vi "LaunchEquations.vi"(7 "Finding V?":bool, 8 "Y (feet)":dbl=8.0, 9 "X (feet)":dbl, 10 "V (m/s)":dbl=14.5, 11 "Angle (degrees)":dbl) -> (2 "V (m/s)":dbl, 3 "Angle (degrees)":dbl)   [LabVIEW 2015]
panel:
  out "Drag (m/s^2)":dbl
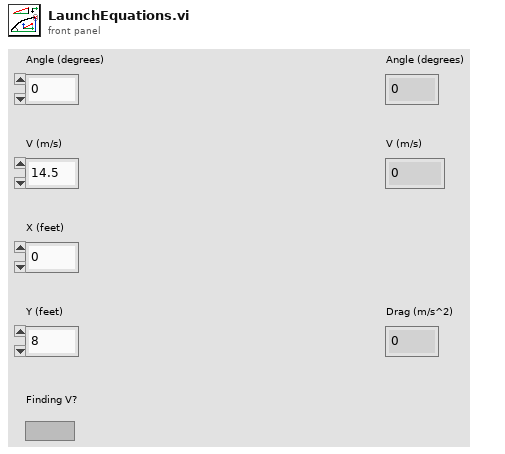
[diagram p1: front panel]
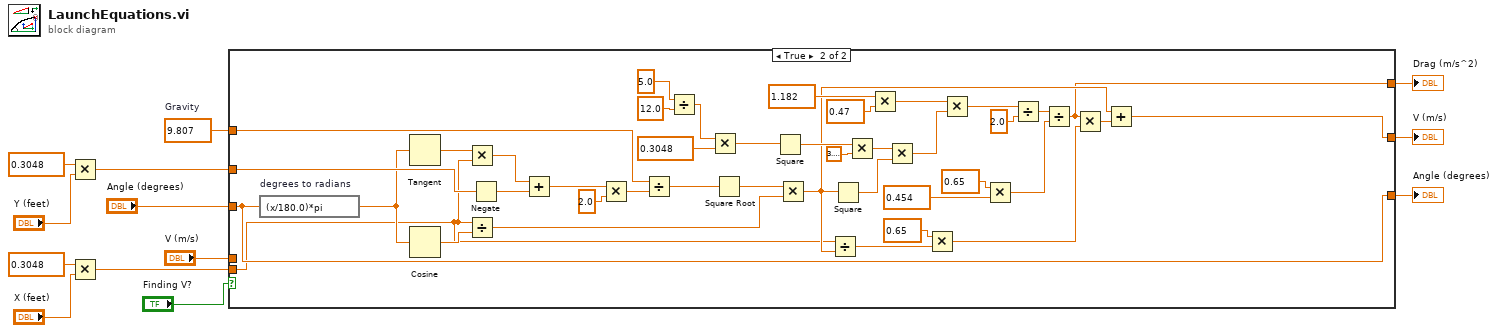
[diagram p0: block diagram]
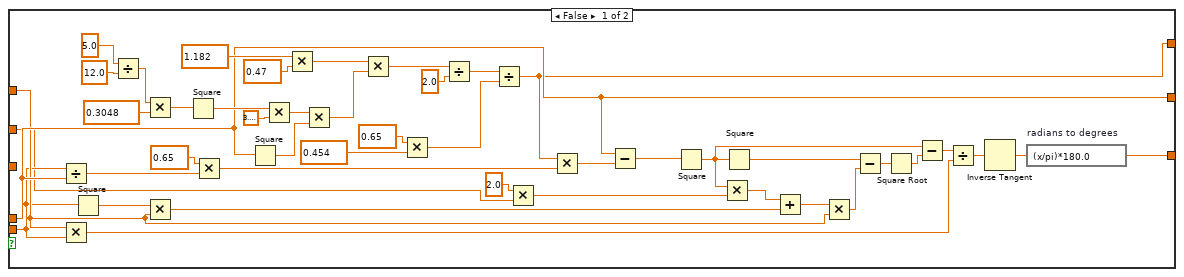
[diagram p2: hidden frame]
diagram:
  w7 = 9.807  # Gravity
  n1 = Multiply(x=0.3048, y="Y (feet)") -> (x*y=w1:dbl)
  n2 = Multiply(x=0.3048, y="X (feet)") -> (x*y=w4:dbl)
  n3 = case shown="True" "Finding V?" {
    tunnel: w4 -> [w16 w60]
    tunnel: "V (m/s)" -> [w18 _]
    tunnel: "Angle (degrees)" -> [_ w89]
    tunnel: [w19 w89] -> w10
    tunnel: [w18 w65] -> w9
    tunnel: [w14 w59] -> w8
    tunnel: w7 -> [w17 w94]
    tunnel: w1 -> [w15 w99]
    frame False {
      n4 = Divide(x=w16, y=w18) -> (x/y=w22:dbl)
      n5 = Multiply(x=w17, y=w16) -> (x*y=w47:dbl)
      n6 = Square(x=w16) -> (x^2=w58:dbl)
      n7 = Divide(x=5.0 ("Radius (in)"), y=12.0 ("Inches-feet")) -> (x/y=w31:dbl)
      n8 = Multiply(x=w31, y=0.3048 ("Feet-meters")) -> (x*y=w30:dbl)
      n9 = Multiply(x=w58, y=w17) -> (x*y=w55:dbl)
      n10 = Square(x=w30) -> (x^2=w42:dbl)
      n11 = Multiply(x=0.65 ("Drag approximation"), y=w22) -> (x*y=w21:dbl)
      n12 = Square(x=w18) -> (x^2=w40:dbl)
      n13 = Multiply(x=w42, y=3.141592653589793) -> (x*y=w41:dbl)
      n14 = Multiply(x=1.182 ("Air density"), y=0.47 ("Drag coefficient")) -> (x*y=w38:dbl)
      n15 = Multiply(x=w41, y=w40) -> (x*y=w39:dbl)
      n16 = Multiply(x=w38, y=w39) -> (x*y=w37:dbl)
      n17 = Multiply(x=0.65 ("Mass (lbs)"), y=0.454 ("Lbs-kgs")) -> (x*y=w26:dbl)
      n18 = Divide(x=w37, y=2.0) -> (x/y=w28:dbl)
      n19 = Divide(x=w28, y=w26) -> (x/y=w14:dbl)
      n20 = Multiply(x=2.0, y=w15) -> (x*y=w56:dbl)
      n21 = Multiply(x=w14, y=w21) -> (x*y=w24:dbl)
      n22 = Subtract(x=w18, y=w24) -> (x-y=w23:dbl)
      n23 = Square(x=w23) -> (x^2=w44:dbl)
      n24 = Multiply(x=w44, y=w56) -> (x*y=w54:dbl)
      n25 = Square(x=w44) -> (x^2=w52:dbl)
      n26 = Add(x=w54, y=w55) -> (x+y=w53:dbl)
      n27 = Multiply(x=w53, y=w17) -> (x*y=w51:dbl)
      n28 = Subtract(x=w52, y=w51) -> (x-y=w50:dbl)
      n29 = Square Root(x=w50) -> (sqrt(x)=w49:dbl)
      n30 = Subtract(x=w44, y=w49) -> (x-y=w48:dbl)
      n31 = Divide(x=w48, y=w47) -> (x/y=w46:dbl)
      n32 = Inverse Tangent(1:w46) -> (0:w45:dbl)
      n33 = expression code="(x/pi)*180.0" "radians to degrees"(w45) -> (w19:dbl)
    }
    frame True {
      n34 = expression code="(x/180.0)*pi" "degrees to radians"(w89) -> (w90:dbl)
      n35 = Tangent(1:w90) -> (0:w91:dbl)
      n36 = Cosine(x=w90) -> (cos(x)=w87:dbl)
      n37 = Multiply(x=w91, y=w60) -> (x*y=w88:dbl)
      n38 = Divide(x=w60, y=w87) -> (x/y=w86:dbl)
      n39 = Negate(x=w99) -> (-x=w98:dbl)
      n40 = Add(x=w88, y=w98) -> (x+y=w96:dbl)
      n41 = Multiply(x=w96, y=2.0) -> (x*y=w95:dbl)
      n42 = Divide(x=w94, y=w95) -> (x/y=w93:dbl)
      n43 = Divide(x=5.0 ("Radius (in)"), y=12.0 ("Inches-feet")) -> (x/y=w74:dbl)
      n44 = Multiply(x=w74, y=0.3048 ("Feet-meters")) -> (x*y=w73:dbl)
      n45 = Square Root(x=w93) -> (sqrt(x)=w92:dbl)
      n46 = Square(x=w73) -> (x^2=w84:dbl)
      n47 = Multiply(x=w92, y=w86) -> (x*y=w61:dbl)
      n48 = Divide(x=w60, y=w61) -> (x/y=w62:dbl)
      n49 = Square(x=w61) -> (x^2=w68:dbl)
      n50 = Multiply(x=w84, y=3.141592653589793) -> (x*y=w83:dbl)
      n51 = Multiply(x=1.182 ("Air density"), y=0.47 ("Drag coefficient")) -> (x*y=w81:dbl)
      n52 = Multiply(x=w83, y=w68) -> (x*y=w82:dbl)
      n53 = Multiply(x=0.65 ("Drag approximation"), y=w62) -> (x*y=w66:dbl)
      n54 = Multiply(x=w81, y=w82) -> (x*y=w80:dbl)
      n55 = Multiply(x=0.65 ("Mass (lbs)"), y=0.454 ("Lbs-kgs")) -> (x*y=w69:dbl)
      n56 = Divide(x=w80, y=2.0) -> (x/y=w71:dbl)
      n57 = Divide(x=w71, y=w69) -> (x/y=w59:dbl)
      n58 = Multiply(x=w59, y=w66) -> (x*y=w64:dbl)
      n59 = Add(x=w61, y=w64) -> (x+y=w65:dbl)
    }
  }
  "V (m/s)" <- w9
  "Angle (degrees)" <- w10
  "Drag (m/s^2)" <- w8
